vi "Beam Profiler Fit Make Image.vi"(8 "Error In":errorcluster, 9 "Pixel Size (µm)":dbl=1.0, 10 "Binning":dbl=1.0, 11 "Image In (U16)":u16[][](array[numeric])) -> (0 "Error Out":errorcluster, 2 "Fit Results":T1, 3 "Fit Image":dbl[][](array[numeric]))   [LabVIEW 2020]
uses:
  Beam Profiler Controls/Beam Profiler Fit Results.ctl
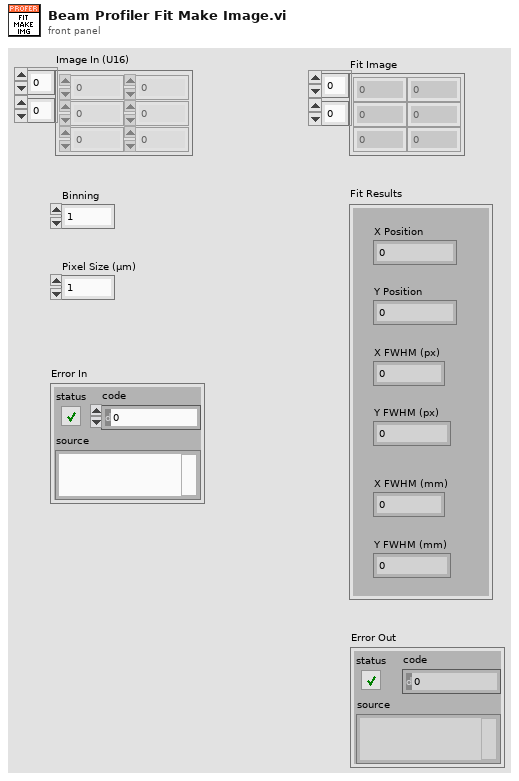
[diagram p1: front panel]
types:
  T1 = typedef "Beam Profiler Fit Results.ctl" = cluster{"X Position":dbl, "Y Position":dbl, "X FWHM (px)":dbl, "Y FWHM (px)":dbl, "X FWHM (mm)":dbl, "Y FWHM (mm)":dbl}
  T2 = typedef "2D Gaussian - Best Fit Parameters.ctl" = cluster{"Amplitude":dbl, "X Position":dbl, "Y Position":dbl, "X Width":dbl, "Y Width":dbl, "Offset":dbl}
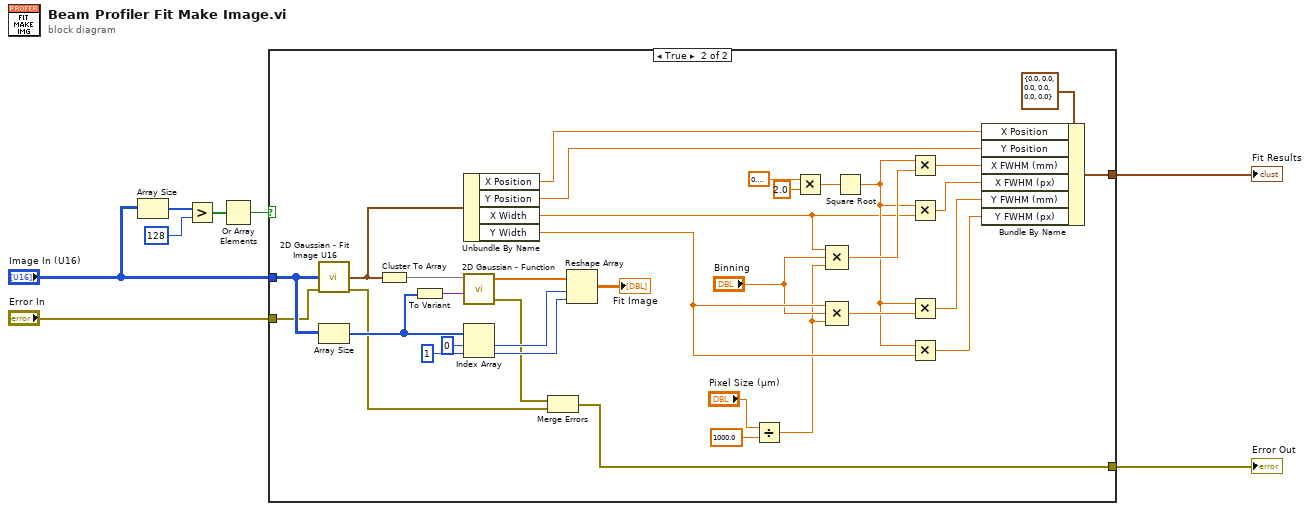
[diagram p0: block diagram]
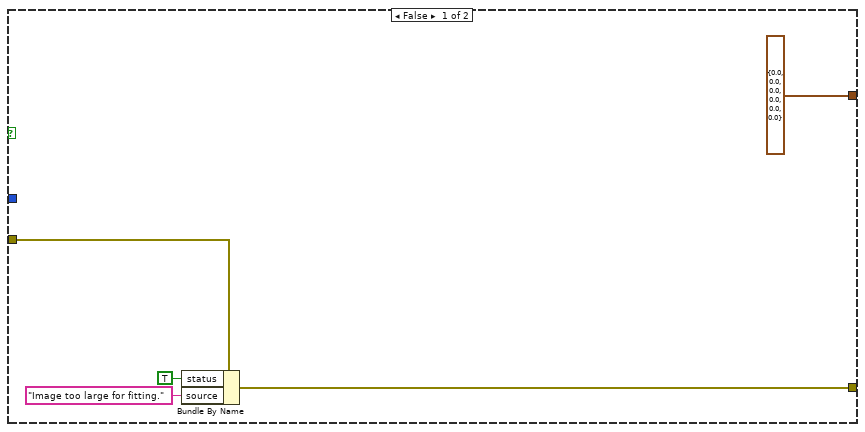
[diagram p2: hidden frame]
diagram:
  n1 = Array Size(array="Image In (U16)") -> (size(s)=w5:i32[])
  n2 = Greater?(x=w5, y=128) -> (0:w3:bool[])
  n3 = Or Array Elements(Boolean array=w3) -> (logical OR=w2:bool)
  n4 = case shown="True" w2 {
    tunnel: "Image In (U16)" -> [_ w29]
    tunnel: [T1 {"X Position"=0.0, "Y Position"=0.0, "X FWHM (px)"=0.0, "Y FWHM (px)"=0.0, "X FWHM (mm)"=0.0, "Y FWHM (mm)"=0.0} ("Fit Results 2") w24] -> w8
    tunnel: [w9 w15] -> w7
    tunnel: "Error In" -> [w12 w14]
    frame False {
      n5 = Bundle By Name(cluster=w12, "status"=TRUE, "source"="Image too large for fitting.") -> (w9:errorcluster)
    }
    frame True {
      n6 = call "2D Gaussian - Fit Image U16.vi"("Image In (U16)"=w29, "Error In"=w14) -> ("Best Fit Params"=w40:T2, "Error Out"=w16:errorcluster)  [unwired: 12 in]
      n7 = Array Size(array=w29) -> (size(s)=w41:i32[])
      n8 = Cluster To Array(cluster=w40) -> (array=w48:dbl[])
      n9 = To Variant(anything=w41) -> (Variant=w42:variant)
      n10 = Unbundle By Name(w40) -> ("X Position"=w19:dbl, "Y Position"=w18:dbl, "X Width"=w31:dbl, "Y Width"=w30:dbl)
      n11 = call "2D Gaussian - Function.vi"("data"=w42, "a"=w48) -> ("error out"=w17:errorcluster, "f(X,a)"=w47:dbl[])  [unwired: 2 in, 1 out]
      n12 = Index Array(array=w41, index #1=0 ("index"), index #2=1 ("index")) -> (element #1=w44:i32, element #2=w43:i32)
      n13 = Merge Errors(w17, w16) -> (w15:errorcluster)
      n14 = Reshape Array(w47, w44, w43) -> (→"Fit Image":dbl[][])
      n15 = Divide(x="Pixel Size (µm)", y=1000.0) -> (x/y=w27:dbl)
      n16 = Multiply(x=0.6931471805599453, y=2.0) -> (x*y=w35:dbl)
      n17 = Compound Arithmetic op=MULTIPLY(w31, "Binning", w27) -> (w33:dbl)
      n18 = Compound Arithmetic op=MULTIPLY(w30, "Binning", w27) -> (w34:dbl)
      n19 = Square Root(x=w35) -> (sqrt(x)=w32:dbl)
      n20 = Multiply(x=w32, y=w33) -> (x*y=w23:dbl)
      n21 = Multiply(x=w32, y=w31) -> (x*y=w22:dbl)
      n22 = Multiply(x=w32, y=w34) -> (x*y=w21:dbl)
      n23 = Multiply(x=w32, y=w30) -> (x*y=w20:dbl)
      n24 = Bundle By Name(cluster=T1 {"X Position"=0.0, "Y Position"=0.0, "X FWHM (px)"=0.0, "Y FWHM (px)"=0.0, "X FWHM (mm)"=0.0, "Y FWHM (mm)"=0.0} ("Fit Results 2"), "X Position"=w19, "Y Position"=w18, "X FWHM (mm)"=w23, "X FWHM (px)"=w22, "Y FWHM (mm)"=w21, "Y FWHM (px)"=w20) -> (w24:T1)
    }
  }
  "Fit Results" <- w8
  "Error Out" <- w7
